vi "Data Pack.vi"(0 "User Information":T3 caption="Informacion del usario" {"Country" items=["Afghanistan", "Aland Islands", "Albania", "Algeria", "American Samoa", "Andorra", "Angola", "Anguilla", "Antarctica", "Antigua And Barbuda", "Argentina", "Armenia", "Aruba", "Australia", "Austria", "Azerbaijan", "Bahamas", "Bahrain", "Bangladesh", "Barbados", "Belarus", "Belgium", "Belize", "Benin", "Bermuda", "Bhutan", "Bolivia", "Bosnia And Herzegovina", "Botswana", "Bouvet Island", "Brazil", "British Indian Ocean Territory", "Brunei Darussalam", "Bulgaria", "Burkina Faso", "Burundi", "Cambodia", "Cameroon", "Canada", "Cape Verde", "Cayman Islands", "Central African Republic", "Chad", "Chile", "China", "Christmas Island", "Cocos (Keeling) Islands", "Colombia", "Comoros", "Congo", "Congo, The Democratic Republic Of The", "Cook Islands", "Costa Rica", "Cote D'Ivoire", "Croatia", "Cuba", "Cyprus", "Czech Republic", "Denmark", "Djibouti", "Dominica", "Dominican Republic", "Ecuador", "Egypt", "El Salvador", "Equatorial Guinea", "Eritrea", "Estonia", "Ethiopia", "Falkland Islands (Malvinas)", "Faroe Islands", "Fiji", "Finland", "France", "French Guiana", "French Polynesia", "French Southern Territories", "Gabon", "Gambia", "Georgia", "Germany", "Ghana", "Gibraltar", "Greece", "Greenland", "Grenada", "Guadeloupe", "Guam", "Guatemala", "Guernsey", "Guinea", "Guinea-Bissau", "Guyana", "Haiti", "Heard Island And Mcdonald Islands", "Holy See (Vatican City State)", "Honduras", "Hong Kong", "Hungary", "Iceland", "India", "Indonesia", "Iran, Islamic Republic Of", "Iraq", "Ireland", "Isle Of Man", "Israel", "Italy", "Jamaica", "Japan", "Jersey", "Jordan", "Kazakhstan", "Kenya", "Kiribati", "Korea, Democratic People'S Republic Of", "Korea, Republic Of", "Kuwait", "Kyrgyzstan", "Lao People'S Democratic Republic", "Latvia", "Lebanon", "Lesotho", "Liberia", "Libyan Arab Jamahiriya", "Liechtenstein", "Lithuania", "Luxembourg", "Macao", "Macedonia, The Former Yugoslav Republic Of", "Madagascar", "Malawi", "Malaysia", "Maldives", "Mali", "Malta", "Marshall Islands", "Martinique", "Mauritania", "Mauritius", "Mayotte", "Mexico", "Micronesia, Federated States Of", "Moldova, Republic Of", "Monaco", "Mongolia", "Montserrat", "Morocco", "Mozambique", "Myanmar", "Namibia", "Nauru", "Nepal", "Netherlands", "Netherlands Antilles", "New Caledonia", "New Zealand", "Nicaragua", "Niger", "Nigeria", "Niue", "Norfolk Island", "Northern Mariana Islands", "Norway", "Oman", "Pakistan", "Palau", "Palestinian Territory, Occupied", "Panama", "Papua New Guinea", "Paraguay", "Peru", "Philippines", "Pitcairn", "Poland", "Portugal", "Puerto Rico", "Qatar", "Reunion", "Romania", "Russian Federation", "Rwanda", "Saint Helena", "Saint Kitts And Nevis", "Saint Lucia", "Saint Pierre And Miquelon", "Saint Vincent And The Grenadines", "Samoa", "San Marino", "Sao Tome And Principe", "Saudi Arabia", "Senegal", "Serbia And Montenegro", "Seychelles", "Sierra Leone", "Singapore", "Slovakia", "Slovenia", "Solomon Islands", "Somalia", "South Africa", "South Georgia And The South Sandwich Islands", "Spain", "Sri Lanka", "Sudan", "Suriname", "Svalbard And Jan Mayen", "Swaziland", "Sweden", "Switzerland", "Syrian Arab Republic", "Taiwan, Province Of China", "Tajikistan", "Tanzania, United Republic Of", "Thailand", "Timor-Leste", "Togo", "Tokelau", "Tonga", "Trinidad And Tobago", "Tunisia", "Turkey", "Turkmenistan", "Turks And Caicos Islands", "Tuvalu", "Uganda", "Ukraine", "United Arab Emirates", "United Kingdom", "United States", "United States Minor Outlying Islands", "Uruguay", "Uzbekistan", "Vanuatu", "Venezuela", "Viet Nam", "Virgin Islands, British", "Virgin Islands, U.S.", "Wallis And Futuna", "Western Sahara", "Yemen", "Zambia", "Zimbabwe", "(Not Specified)"]}, 1 "Project Info":T1 caption="Informacion del proyecto", 3 "Design Inputs":T2={"Q.Plant"=0.05, "C.CoagDoseMax"=0.01, "C.CoagStock"=0.01, "Ti.CoagStock"=0.0015, "EN.DrillSeries"=enum."English", "EN.TubeSeries"=enum."English", "N.SedTanks"=10.0, "N.SedBaysEst"=120.0, "W.SedPlate"=0.005, "L.SedPlateSheet"=0.0, "T.SedPlate"=388800000.0, "T.PlantWall"=0.03, "H.FlocOption"=0.01, "T.FlocBaffleRigidH"=0.03, "T.ConcreteMin"=0.3, "T.SedWeir"=0.3, "T.FlocBaffleRigidV"=108000.0} caption="Datos Basicos" {"T.FlocBaffleRigidV" min=0.0 max=0.2 step=0.001 format="%#.1f"; "T.SedWeir" min=0.001 max=0.2 step=0.001 format="%#.1f"; "T.SedPlate" min=0.001 max=0.05 step=0.001 format="%#.1f"; "T.FlocBaffleRigidH" min=0.0 max=0.2 step=0.001 format="%#.1f"; "T.ConcreteMin" min=0.005 max=0.2 step=0.001 format="%#.1f"; "L.SedPlateSheet" min=0.3 max=8.0 step=0.01 format="%#.1f"; "N.SedBaysEst" min=1.0 max=20.0 step=1.0 format="%#.0f"; "N.SedTanks" min=1.0 max=20.0 step=1.0 format="%#.0f"; "Ti.CoagStock" min=43200.0 max=360000.0 step=3600.0 format="%#.1f"; "H.FlocOption" min=0.5 max=4.0 step=0.01 format="%#.2f"; "C.CoagStock" min=50.0 max=500.0 step=1.0 format="%#.0f"; "C.CoagDoseMax" min=0.03 max=0.2 step=0.005 format="%#.0f"; "Q.Plant" min=0.001 max=0.2 step=0.0001 format="%#.1f"; "T.PlantWall" min=0.05 max=0.5 step=0.001 format="%#.1f"; "W.SedPlate" min=0.5 max=3.0 step=0.001 format="%#.1f"}, 5 "error in":errorcluster, 6 "Packed In":T7, 7 "ADT version":i32, 8 "ADT Commands":T6, 11 "Data transform":enum16{"Pack", "UnPack"}(ring)) -> (10 "ADT Commands out":T6, 12 "Packed Out":T7, 13 "ADT version out":i32, 14 "User Information out":T3 caption="Informacion del usario" {"Country" items=["Afghanistan", "Aland Islands", "Albania", "Algeria", "American Samoa", "Andorra", "Angola", "Anguilla", "Antarctica", "Antigua And Barbuda", "Argentina", "Armenia", "Aruba", "Australia", "Austria", "Azerbaijan", "Bahamas", "Bahrain", "Bangladesh", "Barbados", "Belarus", "Belgium", "Belize", "Benin", "Bermuda", "Bhutan", "Bolivia", "Bosnia And Herzegovina", "Botswana", "Bouvet Island", "Brazil", "British Indian Ocean Territory", "Brunei Darussalam", "Bulgaria", "Burkina Faso", "Burundi", "Cambodia", "Cameroon", "Canada", "Cape Verde", "Cayman Islands", "Central African Republic", "Chad", "Chile", "China", "Christmas Island", "Cocos (Keeling) Islands", "Colombia", "Comoros", "Congo", "Congo, The Democratic Republic Of The", "Cook Islands", "Costa Rica", "Cote D'Ivoire", "Croatia", "Cuba", "Cyprus", "Czech Republic", "Denmark", "Djibouti", "Dominica", "Dominican Republic", "Ecuador", "Egypt", "El Salvador", "Equatorial Guinea", "Eritrea", "Estonia", "Ethiopia", "Falkland Islands (Malvinas)", "Faroe Islands", "Fiji", "Finland", "France", "French Guiana", "French Polynesia", "French Southern Territories", "Gabon", "Gambia", "Georgia", "Germany", "Ghana", "Gibraltar", "Greece", "Greenland", "Grenada", "Guadeloupe", "Guam", "Guatemala", "Guernsey", "Guinea", "Guinea-Bissau", "Guyana", "Haiti", "Heard Island And Mcdonald Islands", "Holy See (Vatican City State)", "Honduras", "Hong Kong", "Hungary", "Iceland", "India", "Indonesia", "Iran, Islamic Republic Of", "Iraq", "Ireland", "Isle Of Man", "Israel", "Italy", "Jamaica", "Japan", "Jersey", "Jordan", "Kazakhstan", "Kenya", "Kiribati", "Korea, Democratic People'S Republic Of", "Korea, Republic Of", "Kuwait", "Kyrgyzstan", "Lao People'S Democratic Republic", "Latvia", "Lebanon", "Lesotho", "Liberia", "Libyan Arab Jamahiriya", "Liechtenstein", "Lithuania", "Luxembourg", "Macao", "Macedonia, The Former Yugoslav Republic Of", "Madagascar", "Malawi", "Malaysia", "Maldives", "Mali", "Malta", "Marshall Islands", "Martinique", "Mauritania", "Mauritius", "Mayotte", "Mexico", "Micronesia, Federated States Of", "Moldova, Republic Of", "Monaco", "Mongolia", "Montserrat", "Morocco", "Mozambique", "Myanmar", "Namibia", "Nauru", "Nepal", "Netherlands", "Netherlands Antilles", "New Caledonia", "New Zealand", "Nicaragua", "Niger", "Nigeria", "Niue", "Norfolk Island", "Northern Mariana Islands", "Norway", "Oman", "Pakistan", "Palau", "Palestinian Territory, Occupied", "Panama", "Papua New Guinea", "Paraguay", "Peru", "Philippines", "Pitcairn", "Poland", "Portugal", "Puerto Rico", "Qatar", "Reunion", "Romania", "Russian Federation", "Rwanda", "Saint Helena", "Saint Kitts And Nevis", "Saint Lucia", "Saint Pierre And Miquelon", "Saint Vincent And The Grenadines", "Samoa", "San Marino", "Sao Tome And Principe", "Saudi Arabia", "Senegal", "Serbia And Montenegro", "Seychelles", "Sierra Leone", "Singapore", "Slovakia", "Slovenia", "Solomon Islands", "Somalia", "South Africa", "South Georgia And The South Sandwich Islands", "Spain", "Sri Lanka", "Sudan", "Suriname", "Svalbard And Jan Mayen", "Swaziland", "Sweden", "Switzerland", "Syrian Arab Republic", "Taiwan, Province Of China", "Tajikistan", "Tanzania, United Republic Of", "Thailand", "Timor-Leste", "Togo", "Tokelau", "Tonga", "Trinidad And Tobago", "Tunisia", "Turkey", "Turkmenistan", "Turks And Caicos Islands", "Tuvalu", "Uganda", "Ukraine", "United Arab Emirates", "United Kingdom", "United States", "United States Minor Outlying Islands", "Uruguay", "Uzbekistan", "Vanuatu", "Venezuela", "Viet Nam", "Virgin Islands, British", "Virgin Islands, U.S.", "Wallis And Futuna", "Western Sahara", "Yemen", "Zambia", "Zimbabwe", "(Not Specified)"]}, 15 "Project Info out":T1 caption="Informacion del proyecto", 16 "user project design":T5, 17 "Design Inputs out":T2={"Q.Plant"=0.05, "C.CoagDoseMax"=0.01, "C.CoagStock"=0.01, "Ti.CoagStock"=0.0015, "EN.DrillSeries"=enum."English", "EN.TubeSeries"=enum."English", "N.SedTanks"=10.0, "N.SedBaysEst"=120.0, "W.SedPlate"=0.005, "L.SedPlateSheet"=0.0, "T.SedPlate"=388800000.0, "T.PlantWall"=0.03, "H.FlocOption"=0.01, "T.FlocBaffleRigidH"=0.03, "T.ConcreteMin"=0.3, "T.SedWeir"=0.3, "T.FlocBaffleRigidV"=108000.0} caption="Datos Basicos" {"T.FlocBaffleRigidV" min=0.0 max=0.2 step=0.001 format="%#.1f"; "T.SedWeir" min=0.001 max=0.2 step=0.001 format="%#.1f"; "T.SedPlate" min=0.001 max=0.05 step=0.001 format="%#.1f"; "T.FlocBaffleRigidH" min=0.0 max=0.2 step=0.001 format="%#.1f"; "T.ConcreteMin" min=0.005 max=0.2 step=0.001 format="%#.1f"; "L.SedPlateSheet" min=0.3 max=8.0 step=0.01 format="%#.1f"; "N.SedBaysEst" min=1.0 max=20.0 step=1.0 format="%#.0f"; "N.SedTanks" min=1.0 max=20.0 step=1.0 format="%#.0f"; "Ti.CoagStock" min=43200.0 max=360000.0 step=3600.0 format="%#.1f"; "H.FlocOption" min=0.5 max=4.0 step=0.01 format="%#.2f"; "C.CoagStock" min=50.0 max=500.0 step=1.0 format="%#.0f"; "C.CoagDoseMax" min=0.03 max=0.2 step=0.005 format="%#.0f"; "Q.Plant" min=0.001 max=0.2 step=0.0001 format="%#.1f"; "T.PlantWall" min=0.05 max=0.5 step=0.001 format="%#.1f"; "W.SedPlate" min=0.5 max=3.0 step=0.001 format="%#.1f"}, 19 "error out":errorcluster)   [LabVIEW 2015]
uses:
  User Information.ctl
  AguaClara Library.lvlib
  Project inputs.ctl
  Basic Inputs.ctl
  ADT Commands.ctl
  packed var.ctl
  user project design.ctl
  Country Ring.ctl
panel:
  in  "Tab Control 2":enum32{"Page 1", "Page 2", "Page 3"}(tab)
  in  "Tab Control":enum32{"Page 1", "Page 2", "Page 3"}(tab)
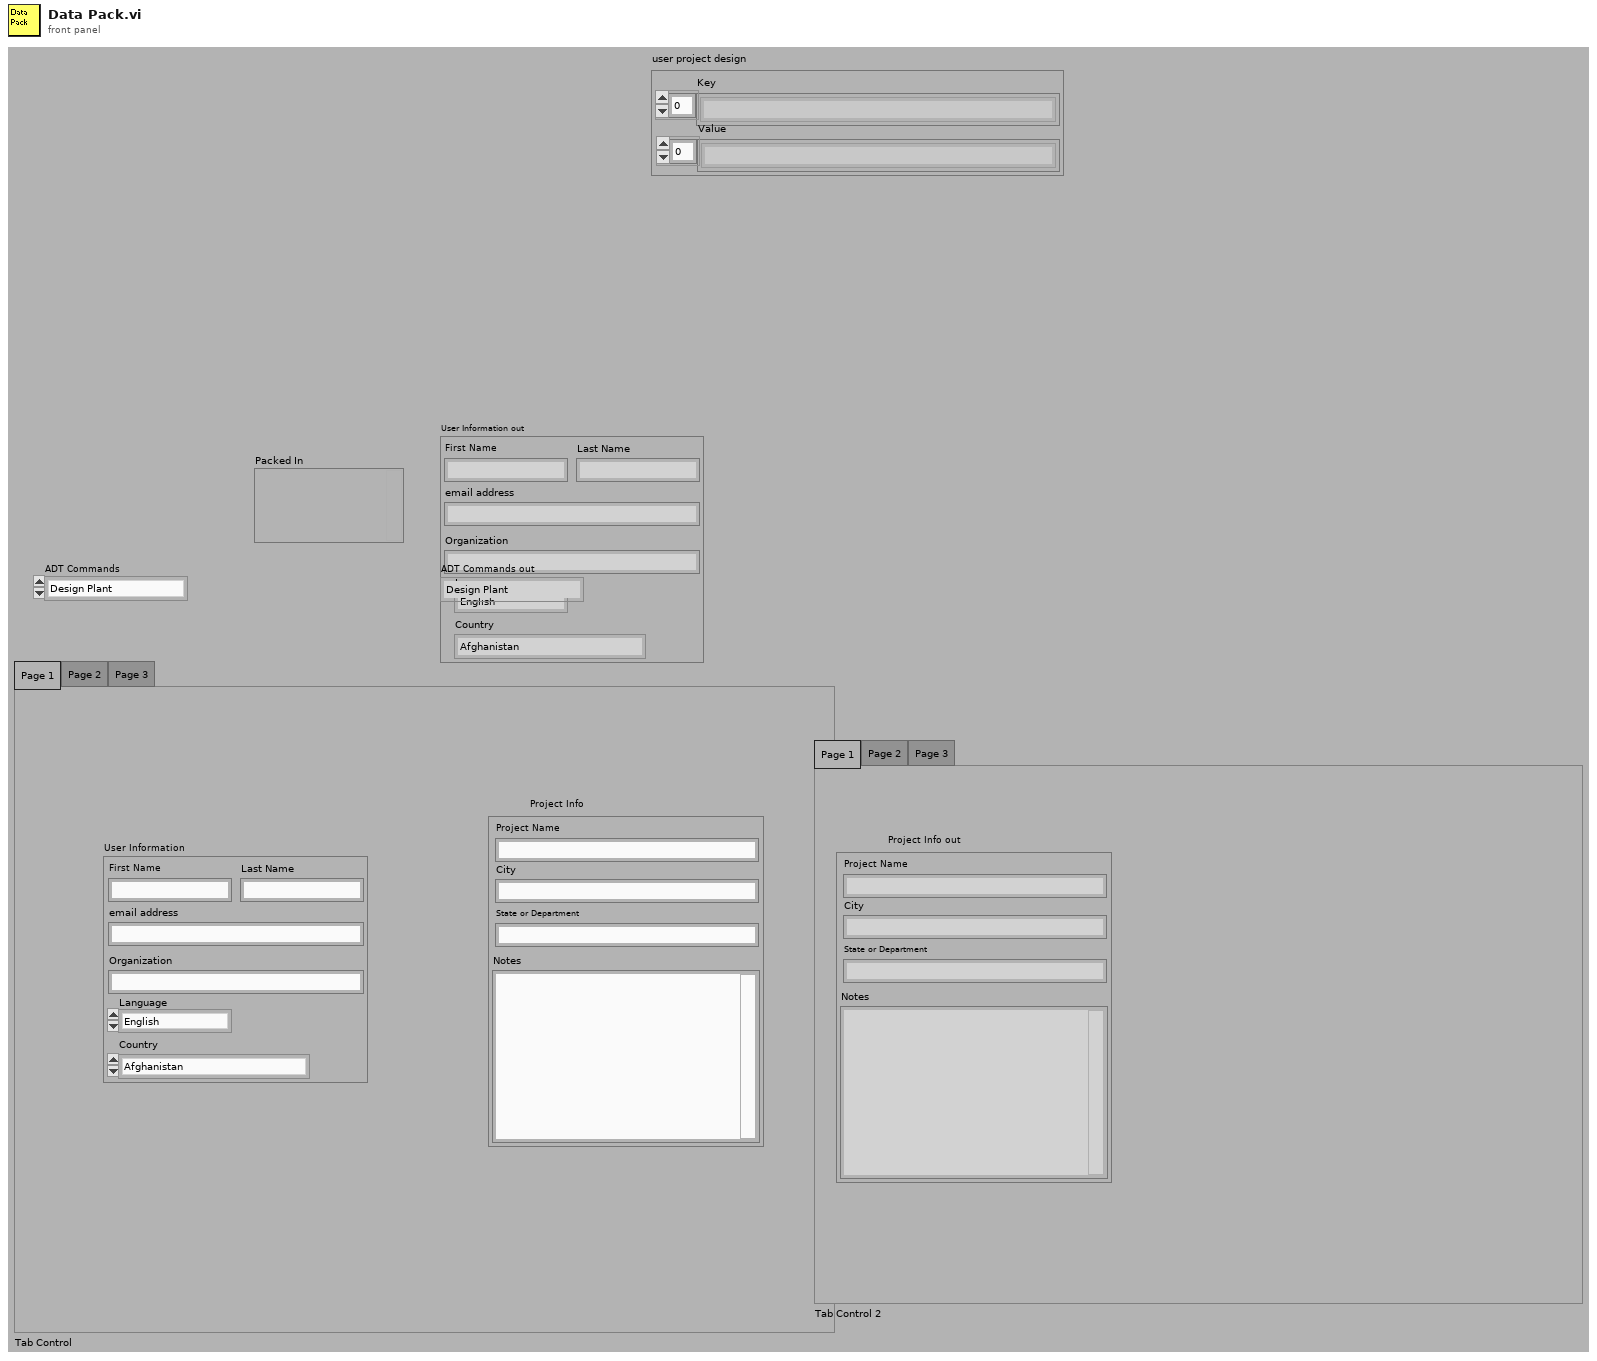
[diagram p1: front panel]
types:
  T1 = typedef "AguaClara Library.lvlib/Project inputs.ctl" = cluster{"Project Name":string, "City":string, "State":string, "Notes":string}
  T2 = typedef "AguaClara Library.lvlib/Basic Inputs.ctl" = cluster{"Q.Plant":dbl[unit], "C.CoagDoseMax":dbl[unit], "C.CoagStock":dbl[unit], "Ti.CoagStock":dbl[unit], "EN.DrillSeries":enum16{"English", "Metric"}, "EN.TubeSeries":enum16{"English", "Metric"}, "N.SedTanks":dbl, "N.SedBaysEst":dbl, "W.SedPlate":dbl[unit], "L.SedPlateSheet":dbl[unit], "T.SedPlate":dbl[unit], "T.PlantWall":dbl[unit], "H.FlocOption":dbl[unit], "T.FlocBaffleRigidH":dbl[unit], "T.ConcreteMin":dbl[unit], "T.SedWeir":dbl[unit], "T.FlocBaffleRigidV":dbl[unit]}
  T3 = typedef "AguaClara Library.lvlib/User Information.ctl" = cluster{"First Name":string, "Last Name":string, "Email Address":string, "Organization":string, "Language":enum16{"English", "Español", "French"}, "Country":T4}
  T4 = typedef "Country Ring.ctl" = u16
  T5 = typedef "user project design.ctl" = cluster{"Key":string[], "Value":string[]}
  T6 = typedef "ADT Commands.ctl" = enum16{"Design Plant", "CheckOut MathCAD Files", "Restart"}
  T7 = typedef "packed var.ctl" = variant
  T8 = cluster{"[0]":variant, "[1]":variant, "[2]":variant, "[3]":variant}
  T9 = cluster{"[0]":variant, "[1]":variant, "[2]":variant}
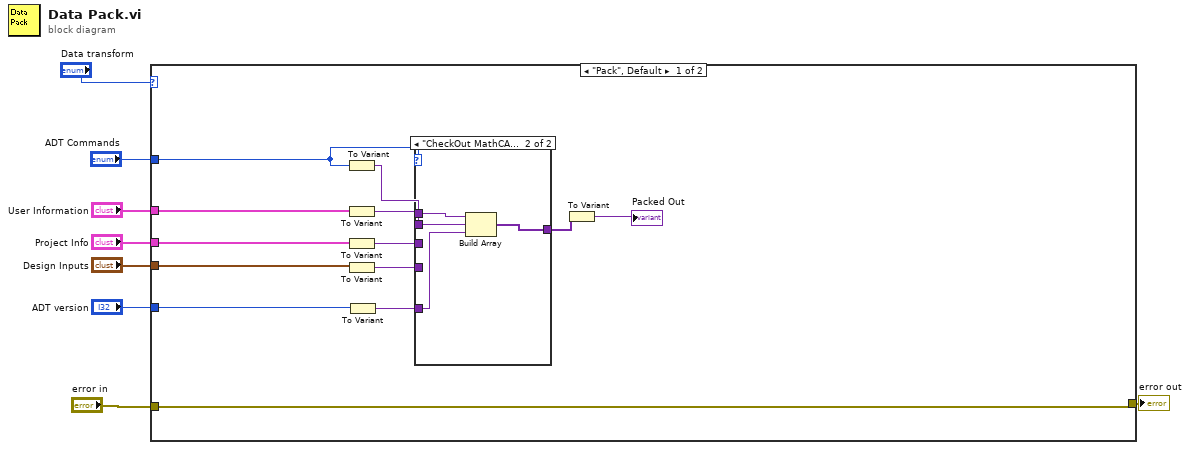
[diagram p0: block diagram]
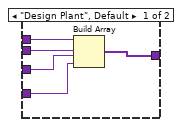
[diagram p2: hidden frame]
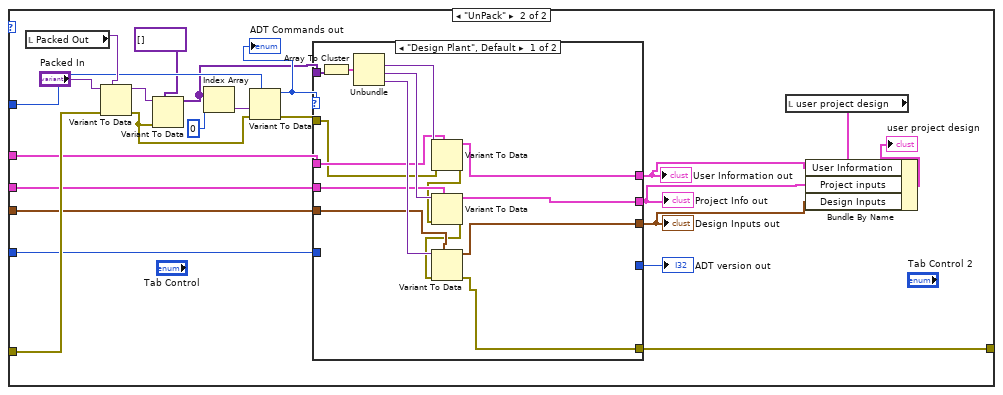
[diagram p3: hidden frame]
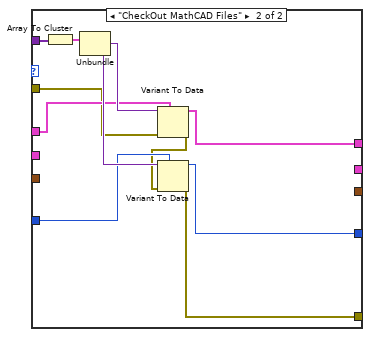
[diagram p4: hidden frame]
diagram:
  n1 = case shown="\"Pack\", Default" "Data transform" {
    tunnel: "error in" -> [w10 w53]
    tunnel: "User Information" -> [w15 w47]
    tunnel: "Project Info" -> [w14 w46]
    tunnel: "Design Inputs" -> [w13 w45]
    tunnel: "ADT version" -> [w12 w44]
    tunnel: "ADT Commands" -> [w11 w48]
    tunnel: [w10 w41] -> w1
    frame "Pack", Default {
      n2 = To Variant(anything=w11) -> (Variant=w21:variant)
      n3 = To Variant(anything=w15) -> (Variant=w20:variant)
      n4 = To Variant(anything=w14) -> (Variant=w19:variant)
      n5 = To Variant(anything=w13) -> (Variant=w18:variant)
      n6 = To Variant(anything=w12) -> (Variant=w16:variant)
      n7 = case shown="\"CheckOut MathCAD Files\"" w11 {
        tunnel: w21 -> [w26 w30]
        tunnel: w20 -> [w25 w29]
        tunnel: w19 -> [w24 _]
        tunnel: w18 -> [w23 _]
        tunnel: [w22 w28] -> w17
        tunnel: w16 -> [_ w27]
        frame "Design Plant", Default {
          n8 = Build Array(w26, w25, w24, w23) -> (w22:variant[])
        }
        frame "CheckOut MathCAD Files" {
          n9 = Build Array(w30, w29, w27) -> (w28:variant[])
        }
      }
      n10 = To Variant(anything=w17) -> (Variant=→"Packed Out":variant)
    }
    frame "UnPack" {
      n11 = local read "Packed Out"() -> (w50:T7)
      n12 = Variant To Data(error in=w53, type=w50, Variant="Packed In") -> (data=w38:T7, error out=w39:errorcluster)
      n13 = Variant To Data(error in=w39, type=variant[] [], Variant=w38) -> (data=w36:variant[])  [unwired: 1 out]
      n14 = Index Array(array=w36, index=0) -> (element=w49:variant)
      n15 = Variant To Data(error in=w39, type=w48, Variant=w49) -> (data=w40:T6, error out=w42:errorcluster)
      "ADT Commands out" <- w40
      n16 = case shown="\"Design Plant\", Default" w40 {
        tunnel: w36 -> [w68 w78]
        tunnel: w47 -> [w63 w75]
        tunnel: w46 -> [w62 _]
        tunnel: w45 -> [w61 _]
        tunnel: [w60 _] -> w31
        tunnel: [w59 _] -> w32
        tunnel: [w58 w72] -> w33
        tunnel: w44 -> [_ w74]
        tunnel: [_ w73] -> w43
        tunnel: w42 -> [w57 w71]
        tunnel: [w54 w69] -> w41
        frame "Design Plant", Default {
          n17 = Array To Cluster(array=w68) -> (cluster=w67:T8)
          n18 = Unbundle(w67) -> ("[1]"=w66:variant, "[2]"=w65:variant, "[3]"=w64:variant)  [unwired: 1 out]
          n19 = Variant To Data(error in=w57, type=w63, Variant=w66) -> (data=w58:T3, error out=w56:errorcluster)
          n20 = Variant To Data(error in=w56, type=w62, Variant=w65) -> (data=w59:T1, error out=w55:errorcluster)
          n21 = Variant To Data(error in=w55, type=w61, Variant=w64) -> (data=w60:T2, error out=w54:errorcluster)
        }
        frame "CheckOut MathCAD Files" {
          n22 = Array To Cluster(array=w78) -> (cluster=w79:T9)
          n23 = Unbundle(w79) -> ("[1]"=w77:variant, "[2]"=w76:variant)  [unwired: 1 out]
          n24 = Variant To Data(error in=w71, type=w75, Variant=w77) -> (data=w72:T3, error out=w70:errorcluster)
          n25 = Variant To Data(error in=w70, type=w74, Variant=w76) -> (data=w73:i32, error out=w69:errorcluster)
        }
      }
      "ADT version out" <- w43
      "User Information out" <- w33
      "Project Info out" <- w32
      "Design Inputs out" <- w31
      n26 = local read "user project design"() -> (w35:T5)
      n27 = Bundle By Name(cluster=w35, "User Information"=w33, "Project inputs"=w32, "Design Inputs"=w31) -> (→"user project design":T5)
    }
  }
  "error out" <- w1
